vi "sphere.vi"(0 "Radius":sgl=1.0) -> (4 "urdf out":string="<cylinder>\n  <radius>1.00</radius>\n  <length>1.00</length>\n</cylinder>")   [LabVIEW 2010]
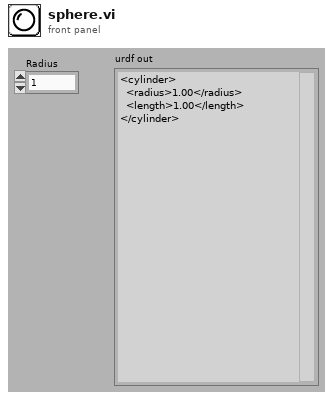
[diagram p1: front panel]
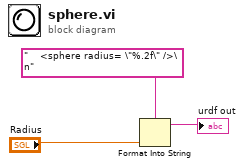
[diagram p0: block diagram]
diagram:
  n1 = Format Into String(format string="    <sphere radius= \"%.2f\" />\n", "Radius") -> (resulting string=→"urdf out":string)  [unwired: 2 in, 1 out]
